vi "AuMT8852B  Close.vi"(8 "error in (no error)":errorcluster, 11 "VISA session":refnum<visa-resource-name>) -> (0 "error out":errorcluster, 2 "error code":i32)   [LabVIEW 2017]
doc: "Anritsu MT8852B Bluetooth Tester\n\nCloses the instrument session and deallocates memory used by the instrument driver."
uses:
  <instrlib>/aumt8852B/General/Utilities/Instrument.llb/Instrument Object Reference.ctl
panel:
  in  "reference":T1
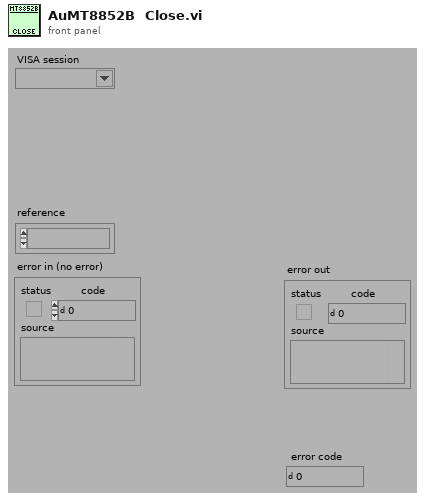
[diagram p1: front panel]
types:
  T1 = typedef "Instrument Object Reference.ctl" = refnum<k1>
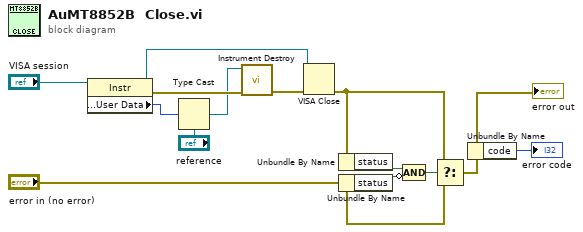
[diagram p0: block diagram]
diagram:
  n1 = property class="Instr"(reference="VISA session") -> (reference out=w11:refnum<visa-resource-name>, error out=w9:errorcluster, "General Settings:User Data"=w12:u32)  [unwired: 1 in]
  n2 = Type Cast(type="reference", x=w12) -> (*(type *) &x=w8:T1)
  n3 = call <instrlib>:"Instrument Destroy.vi"("error in (no error)"=w9, "reference"=w8) -> ("error out"=w10:errorcluster)  [unwired: 5 in]
  n4 = VISA Close(VISA resource name=w11, error in (no error)=w10) -> (error out=w4:errorcluster)
  n5 = Unbundle By Name(w4) -> ("status"=w3:bool)
  n6 = Unbundle By Name("error in (no error)") -> ("status"=w2:bool)
  n7 = Compound Arithmetic op=AND(w3, invert w2) -> (w1:bool)
  n8 = Select(t=w4, s=w1, f="error in (no error)") -> (s? t:f=w5:errorcluster)
  "error out" <- w5
  n9 = Unbundle By Name(w5) -> ("code"=→"error code":i32)
